vi "Main.vi"() -> ()   [LabVIEW 2020]
doc: "This template is for the Queued Message Handler design pattern.\n\nThe Event Handling Loop generates messages based on user interface actions.\n\nThe Message Handling Loop processes messages generated by the Event Handling Loop, or by other messages. The messages are string values, so new messages can be added easily to the Message Cases case structure in the Message Handling Loop. Each message cluster can also provide an optional value for Message Data, which is a variant that can be converted to whatever message-specific data is required."
uses:
  controls/UI Data.ctl
  support/Message Queue/Enqueue Message (Single).vi
  <vilib>/Utility/error.llb/Error Cluster From Error Code.vi
  <vilib>/ErrorRing/Error Ring.xnode
  support/Message Queue/Message Queue.lvlib
  support/User Event - Stop/User Event - Stop.lvlib
panel:
  out "Status":bool
  out "Wybrany zakres f":string
  in  "Pojemnik":enum32{"Page 1", "Page 2"}(tab)
  in  "Kondensator 1":bool
  in  "Kondensator 2":bool
  in  "Kondensator 3":bool
  in  "Kondensator 4":bool
  in  "Cewka":bool
  in  "Cewki":enum32{"Cewki", "Page 2"}(tab)
  in  "L1":bool
  in  "L2":bool
  in  "L 3":bool
  in  "L 4":bool
  in  "Zakres Q":u8(knob) scale=0.0..10.0
  in  "C_reg2":dbl(knob) scale=-5.0..5.0
  in  "Zakres f":u8(knob) scale=0.0..6.0
  in  "ON/OFF":bool
  out "Dobroæ":dbl(knob) scale=0.0..50.0
  in  "C_reg":dbl(knob) scale=520.0..30.0
  in  "Czêstotliwoœæ":dbl(knob) min=3.0 max=950.0 scale=950.0..1045.0
  in  "Exit":bool
  # "Q"
  # "f"
  # "C (pF)"
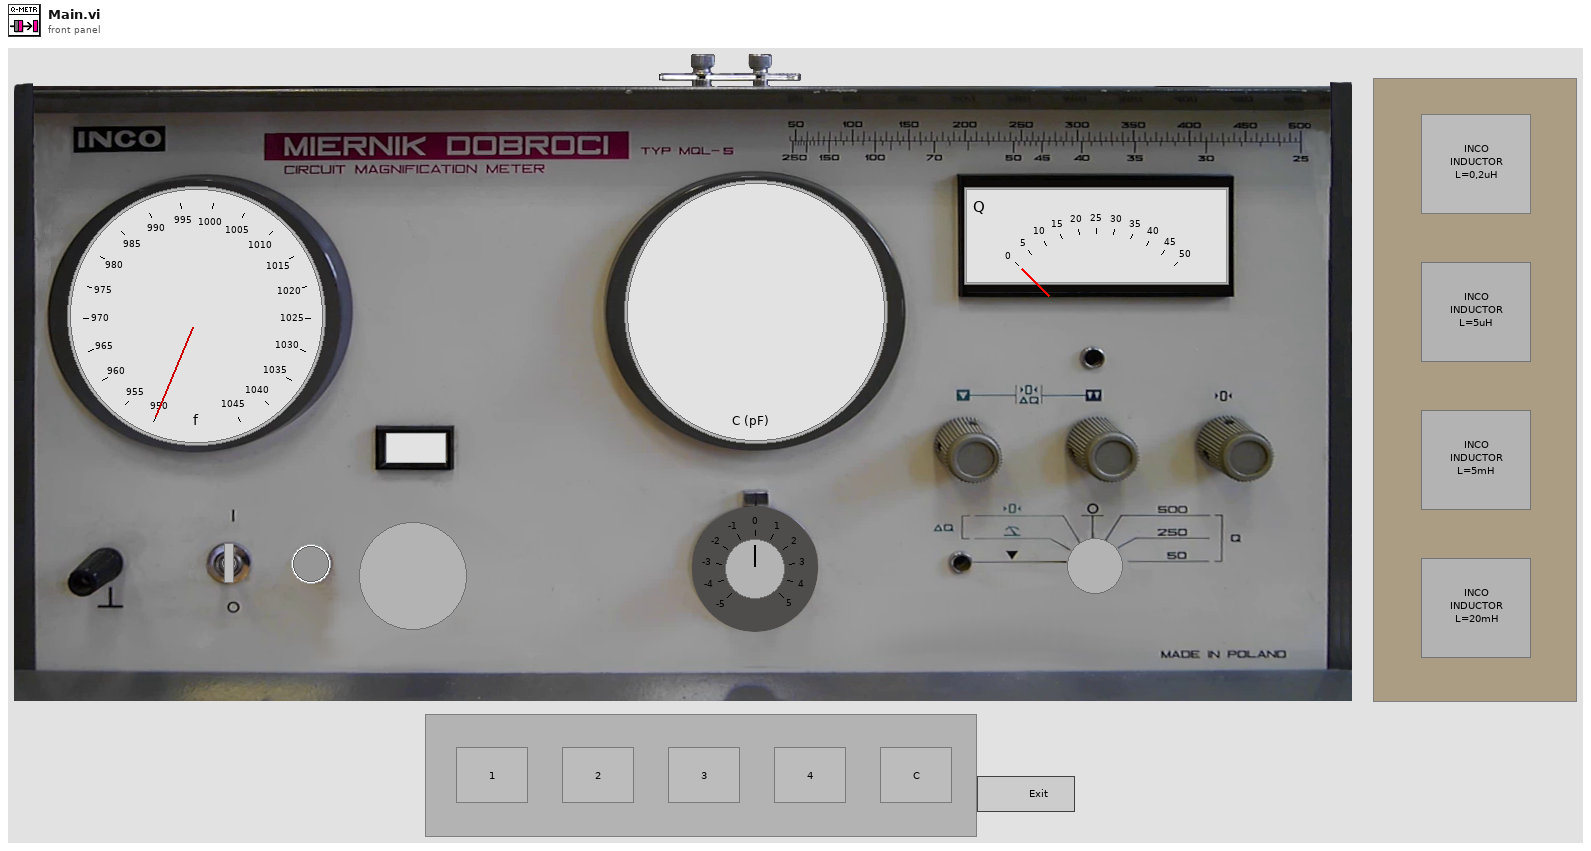
[diagram p1: front panel]
types:
  T1 = typedef "UI Data.ctl" = cluster{"Zakres freq":u8, "Status":bool, "C_reg":dbl, "C_reg2":dbl, "L1":bool, "L2":bool, "L3":bool, "L4":bool, "L value":dbl, "C1":bool, "C2":bool, "C3":bool, "C4":bool, "C measure":dbl, "Freq":dbl, "Q elementu":dbl, "L cewka":bool, "C prev":dbl, "C byl zamon.":bool, "Q prev":dbl}
  T2 = typedef "Message Queue.lvlib/All Message Queues.ctl" = cluster{"UI":refnum<queue>}
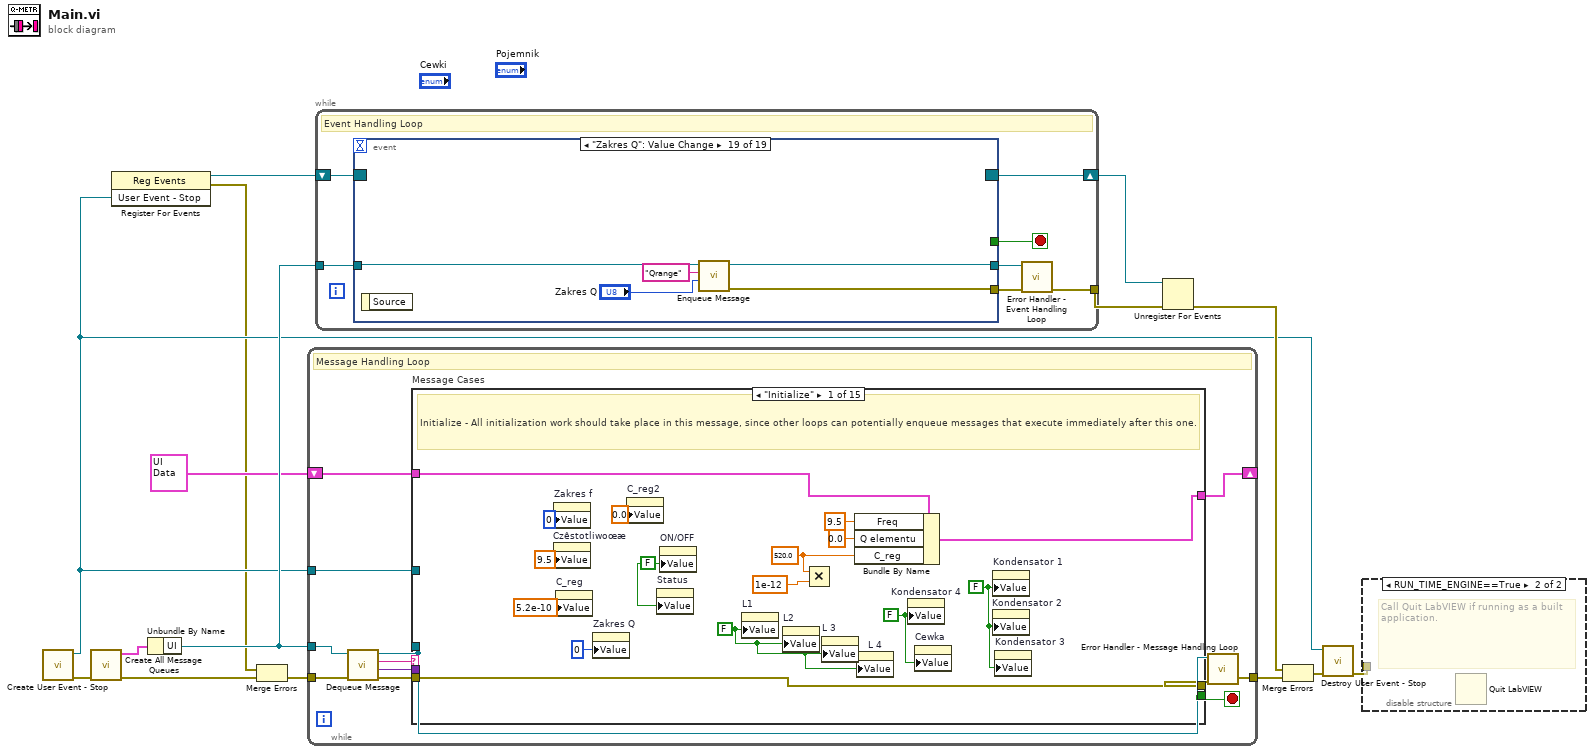
[diagram p0: block diagram]
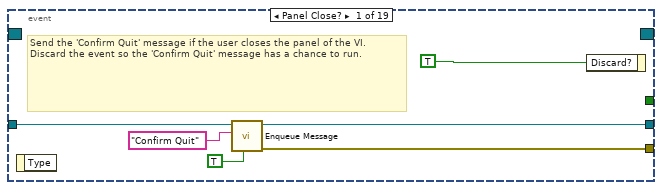
[diagram p3: hidden frame]
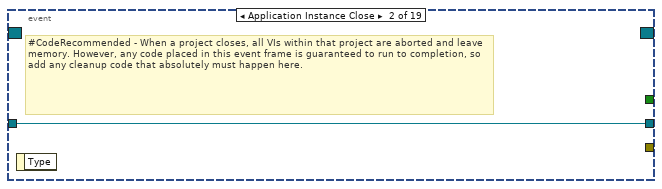
[diagram p4: hidden frame]
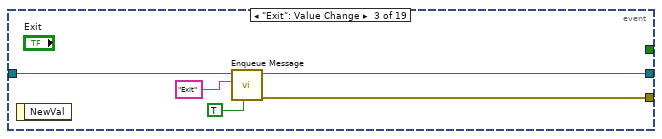
[diagram p5: hidden frame]
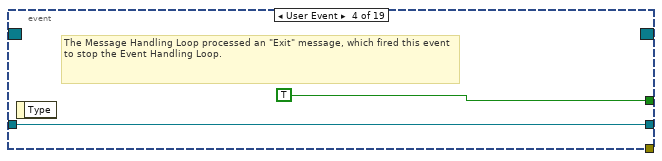
[diagram p6: hidden frame]
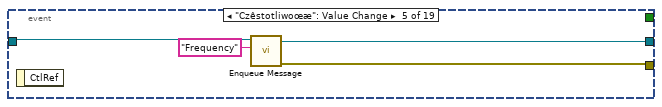
[diagram p7: hidden frame]
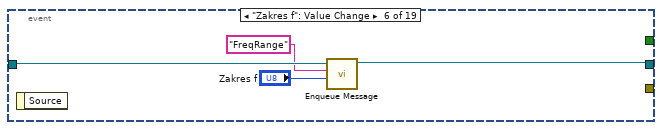
[diagram p8: hidden frame]
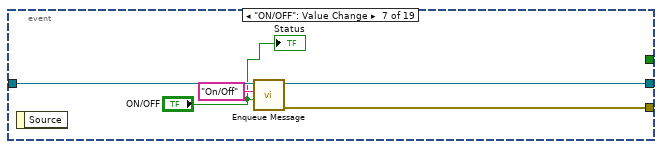
[diagram p9: hidden frame]
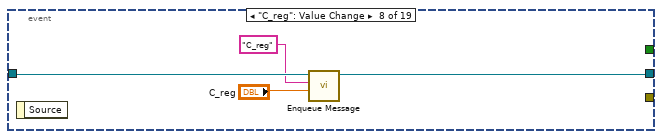
[diagram p10: hidden frame]
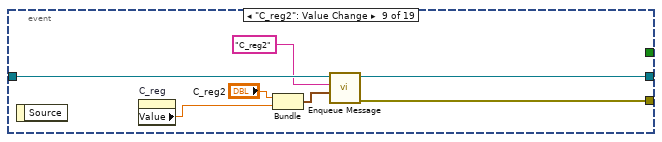
[diagram p11: hidden frame]
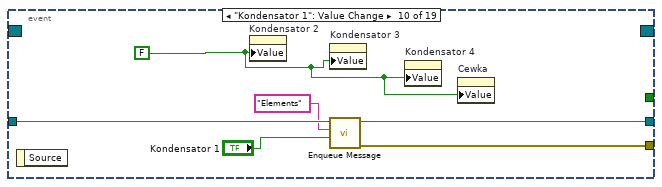
[diagram p12: hidden frame]
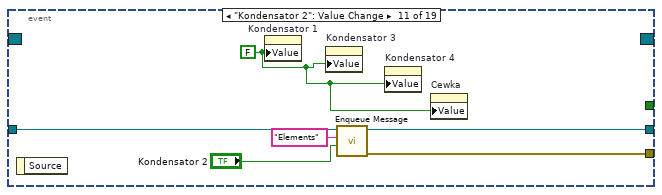
[diagram p13: hidden frame]
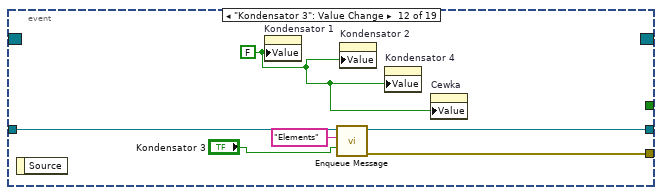
[diagram p14: hidden frame]
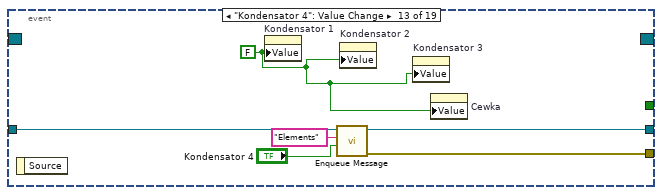
[diagram p15: hidden frame]
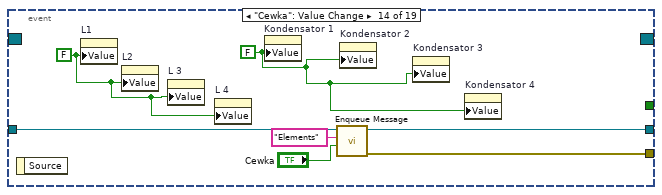
[diagram p16: hidden frame]
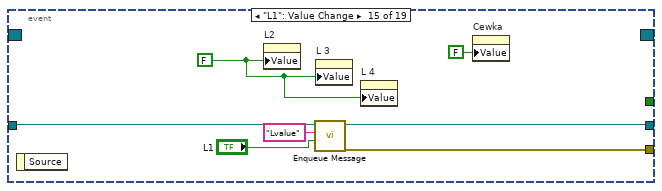
[diagram p17: hidden frame]
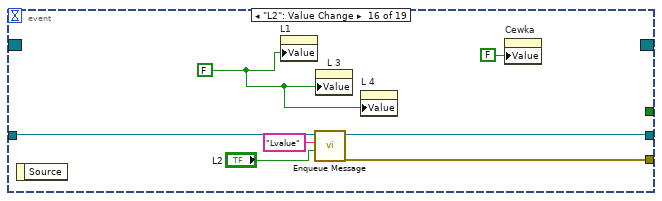
[diagram p18: hidden frame]
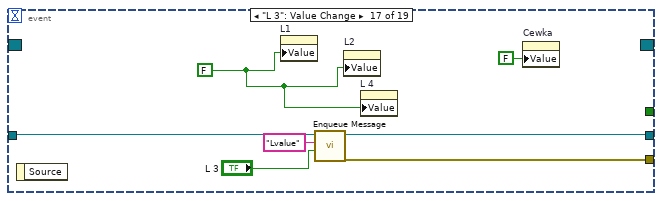
[diagram p19: hidden frame]
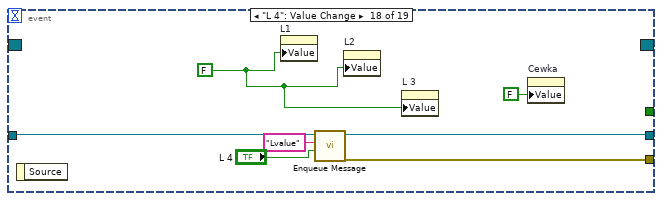
[diagram p20: hidden frame]
diagram:
  n1 = call "Create User Event - Stop.vi"() -> ("error out"=w11:errorcluster, "User Event - Stop"=w3:refnum<user-event>)  [unwired: 10 in]
  n2 = call "Create All Message Queues.vi"("error in (no error)"=w11) -> ("error out"=w15:errorcluster, "Message Queues out"=w14:T2)  [unwired: 9 in]
  n3 = register-events(w3) -> (reference out=w4:refnum<event-registration>, error out=w1:errorcluster)  [unwired: 2 in]
  n4 = Unbundle By Name(w14) -> ("UI"=w12:refnum<queue>)
  n5 = Merge Errors(w1, w15) -> (w2:errorcluster)
  n6 = while {
    tunnel: w12 -> [w20]
    shift-right: [w27] -> _
    shift-left: T1 {"Zakres freq"=0, "Status"=FALSE, "C_reg"=0.0, "C_reg2"=0.0, "L1"=FALSE, "L2"=FALSE, "L3"=FALSE, "L4"=FALSE, "L value"=0.0, "C1"=FALSE, "C2"=FALSE, "C3"=FALSE, "C4"=FALSE, "C measure"=0.0, "Freq"=0.0, "Q elementu"=0.0, "L cewka"=FALSE, "C prev"=0.0, "C byl zamon."=FALSE, "Q prev"=0.0} ("Data Cluster") -> [w16]
    tunnel: w3 -> [w25]
    tunnel: w2 -> [w24]
    tunnel: [w18] -> w13
    stop <- w26 stop-if-true
    # "Message Handling Loop"
    n7 = call "Dequeue Message.vi"("error in (no error)"=w24, "Message Queue"=w20) -> ("error out"=w23:errorcluster, "Message Data"=w21:variant, "Message"=w22:string, "dup Message Queue"=w19:refnum<queue>)  [unwired: 6 in]
    n8 = case "Message Cases" shown="\"Initialize\"" w22 {
      selector: w22 -> [_ _ _ _ _ _ _ _ _ _ _ _ _ _ w264]
      tunnel: w19 -> [_ _ w53 _ w66 w80 w110 w163 w175 w188 w218 w233 _ w263 _]
      tunnel: w23 -> [w43 w50 w57 w60 w68 w79 w111 w165 w177 w186 w217 w235 w252 w256 _]
      tunnel: [w43 w44 w55 w58 w69 w81 w113 w166 w178 w189 w220 w236 w251 w259 w265] -> w17
      tunnel: w16 -> [w37 w49 w56 w59 w70 w76 w107 w157 w171 w182 w216 w229 w250 w262 w266]
      tunnel: [w36 w49 w56 w59 w70 w75 w106 w161 w170 w180 w216 w228 w250 w262 w266] -> w27
      tunnel: [_ _ _ _ _ _ _ _ _ _ _ _ _ TRUE _] -> w26
      tunnel: w21 -> [_ w48 _ _ w64 _ _ w160 w173 w184 _ _ _ w253 _]
      tunnel: w25 -> [_ _ _ _ _ _ _ _ _ _ _ _ _ w258 _]
      frame "Initialize" {
        w29 = FALSE ("L1")
        w30 = FALSE ("Kondensator 4")
        w31 = FALSE ("Kondensator 1")
        w33 = 520.0 ("C_reg")
        w38 = FALSE ("ON/OFF")
        # "Initialize - All initialization work should take place in this message, since other loops can potentially enqueue messages that execute immediately after this one."
        n9 = property on="Zakres f" class="Knob (strict)"("Value"=u8 0 ("Zakres f")) -> ()  [unwired: 2 in, 2 out]
        n10 = property on="Czêstotliwoœæ" class="Knob (strict)"("Value"=9.5 ("Czêstotliwoœæ")) -> ()  [unwired: 2 in, 2 out]
        n11 = property on="C_reg" class="Knob (strict)"("Value"=5.2e-10 ("C_reg")) -> ()  [unwired: 2 in, 2 out]
        n12 = property on="Zakres Q" class="Knob (strict)"("Value"=u8 0 ("Zakres Q")) -> ()  [unwired: 2 in, 2 out]
        n13 = property on="C_reg2" class="Knob (strict)"("Value"=0.0 ("C_reg2")) -> ()  [unwired: 2 in, 2 out]
        n14 = property on="Status" class="Bool (strict)"("Value"=w38) -> ()  [unwired: 2 in, 2 out]
        n15 = property on="ON/OFF" class="Bool (strict)"("Value"=w38) -> ()  [unwired: 2 in, 2 out]
        n16 = property on="L1" class="Bool (strict)"("Value"=w29) -> ()  [unwired: 2 in, 2 out]
        n17 = property on="L2" class="Bool (strict)"("Value"=w29) -> ()  [unwired: 2 in, 2 out]
        n18 = Multiply(x=w33, y=1e-12) -> ()  [unwired: 1 out]
        n19 = property on="L 3" class="Bool (strict)"("Value"=w29) -> ()  [unwired: 2 in, 2 out]
        n20 = Bundle By Name(cluster=w37, "Freq"=9.5, "Q elementu"=0.0, "C_reg"=w33) -> (w36:T1)
        n21 = property on="L 4" class="Bool (strict)"("Value"=w29) -> ()  [unwired: 2 in, 2 out]
        n22 = property on="Kondensator 4" class="Bool (strict)"("Value"=w30) -> ()  [unwired: 2 in, 2 out]
        n23 = property on="Cewka" class="Bool (strict)"("Value"=w30) -> ()  [unwired: 2 in, 2 out]
        n24 = property on="Kondensator 1" class="Bool (strict)"("Value"=w31) -> ()  [unwired: 2 in, 2 out]
        n25 = property on="Kondensator 2" class="Bool (strict)"("Value"=w31) -> ()  [unwired: 2 in, 2 out]
        n26 = property on="Kondensator 3" class="Bool (strict)"("Value"=w31) -> ()  [unwired: 2 in, 2 out]
      }
      frame "Error" {
        # "#CodeRecommended - If you ever change the name of this \"Error\" message, you'll need to update the name in the Check Loop Error.vi as well."
        # "#CodeRecommended - Consider creating a system for logging errors in some way. These errors are for notification purposes only. Handling of specific errors should be performed in the message frames that generated the error."
        # "Error - Display an error dialog. This message is sent by the \"Error Handler\" VIs at the end of other loops in this application."
        n27 = Variant To Data(error in=w50, type=errorcluster {"status"=FALSE, "code"=0, "source"=""} ("error constant"), Variant=w48) -> (data=w46:errorcluster, error out=w45:errorcluster)
        n28 = call <vilib>:"Simple Error Handler.vi"("error in (no error)"=w46) -> ()  [unwired: 4 in, 5 out]
        n29 = Merge Errors(w45) -> (w44:errorcluster)
      }
      frame "Confirm Quit" {
        # "#CodeNeeded - If you want to provide an \"Are you sure\" dialog (or some other notification) before the application exits, place that code here. This message is typically sent from a Panel Close? event."
        # "Confirm Quit - Message that can confirm whether or not the user wants to exit the application."
        n30 = call-poly "Enqueue Message.vi"("Priority Message? (F)"=TRUE, "error in (no error)"=w57, "Message"="Exit", "Message Queue"=w53) -> ("error out"=w54:errorcluster)  [unwired: 6 in, 1 out]
        n31 = Merge Errors(w54) -> (w55:errorcluster)
      }
      frame "---Copy This Frame---" {
        # "Duplicate this frame when creating new messages.  Change this comment in the duplicated frame to describe this message."
        n32 = Merge Errors(w60) -> (w58:errorcluster)
      }
      frame "Qrange" {
        # "Duplicate this frame when creating new messages.  Change this comment in the duplicated frame to describe this message."
        n33 = Variant To Data(type=u8 0 ("Zakres Q"), Variant=w64) -> (data=w62:u8)  [unwired: 1 in, 1 out]
        n34 = call-poly "Enqueue Message.vi"("error in (no error)"=w68, "Message"="On/Off", "Message Queue"=w66) -> ("error out"=w67:errorcluster)  [unwired: 7 in, 1 out]
        n35 = case shown="8.." w62 {
          tunnel: [500.0 ("Scale.Range:Maximum") 250.0 ("Scale.Range:Maximum") 50.0 ("Scale.Range:Maximum")] -> w61
          frame 0..6, Default {
          }
          frame 7 {
          }
          frame 8.. {
          }
        }
        n36 = property on="Dobroæ" class="Knob (strict)"("Scale.Maximum"=w61) -> ()  [unwired: 2 in, 2 out]
        n37 = Merge Errors(w67) -> (w69:errorcluster)
      }
      frame "Lvalue" {
        # "Duplicate this frame when creating new messages.  Change this comment in the duplicated frame to describe this message."
        n38 = property on="L1" class="Bool (strict)"() -> ("Value"=w74:bool)  [unwired: 2 in, 2 out]
        n39 = call-poly "Enqueue Message.vi"("error in (no error)"=w79, "Message"="On/Off", "Message Queue"=w80) -> ("error out"=w78:errorcluster)  [unwired: 7 in, 1 out]
        n40 = case shown="False" w74 {
          tunnel: w76 -> [w83 w105]
          tunnel: [w82 w104] -> w75
          frame False {
            n41 = property on="L2" class="Bool (strict)"() -> ("Value"=w84:bool)  [unwired: 2 in, 2 out]
            n42 = case shown="False" w84 {
              tunnel: w83 -> [w86 w102]
              tunnel: [w85 w101] -> w82
              frame False {
                n43 = property on="L 3" class="Bool (strict)"() -> ("Value"=w87:bool)  [unwired: 2 in, 2 out]
                n44 = case shown="False" w87 {
                  tunnel: w86 -> [w89 w99]
                  tunnel: [w88 w98] -> w85
                  frame False {
                    n45 = property on="L 4" class="Bool (strict)"() -> ("Value"=w90:bool)  [unwired: 2 in, 2 out]
                    n46 = case shown="False" w90 {
                      tunnel: w89 -> [w93 w96]
                      tunnel: [w92 w95] -> w88
                      frame False {
                        n47 = Bundle By Name(cluster=w93, "L value"=0.0) -> (w92:T1)
                      }
                      frame True {
                        n48 = Bundle By Name(cluster=w96, "L value"=0.02) -> (w95:T1)
                      }
                    }
                  }
                  frame True {
                    n49 = Bundle By Name(cluster=w99, "L value"=0.005) -> (w98:T1)
                  }
                }
              }
              frame True {
                n50 = Bundle By Name(cluster=w102, "L value"=5e-06) -> (w101:T1)
              }
            }
          }
          frame True {
            n51 = Bundle By Name(cluster=w105, "L value"=2e-07) -> (w104:T1)
          }
        }
        n52 = Merge Errors(w78) -> (w81:errorcluster)
      }
      frame "Elements" {
        # "Duplicate this frame when creating new messages.  Change this comment in the duplicated frame to describe this message."
        n53 = property on="Kondensator 1" class="Bool (strict)"() -> ("Value"=w108:bool)  [unwired: 2 in, 2 out]
        n54 = case shown="True" w108 {
          tunnel: w107 -> [w115 w149]
          tunnel: [w114 w148] -> w106
          frame False {
            n55 = property on="Kondensator 2" class="Bool (strict)"() -> ("Value"=w116:bool)  [unwired: 2 in, 2 out]
            n56 = case shown="True" w116 {
              tunnel: w115 -> [w119 w145]
              tunnel: [w118 w144] -> w114
              frame False {
                n57 = property on="Kondensator 3" class="Bool (strict)"() -> ("Value"=w117:bool)  [unwired: 2 in, 2 out]
                n58 = case shown="False" w117 {
                  tunnel: w119 -> [w121 w141]
                  tunnel: [w120 w140] -> w118
                  frame False {
                    n59 = property on="Kondensator 4" class="Bool (strict)"() -> ("Value"=w122:bool)  [unwired: 2 in, 2 out]
                    n60 = case shown="False" w122 {
                      tunnel: w121 -> [w124 w137]
                      tunnel: [w123 w136] -> w120
                      frame False {
                        n61 = property on="Cewka" class="Bool (strict)"() -> ("Value"=w125:bool)  [unwired: 2 in, 2 out]
                        n62 = case shown="False" w125 {
                          tunnel: w124 -> [w128 w133]
                          tunnel: [w129 w132] -> w123
                          frame False {
                            n63 = Bundle By Name(cluster=w128, "Q elementu"=0.0, "C measure"=0.0) -> (w129:T1)
                          }
                          frame True {
                            n64 = Bundle By Name(cluster=w133, "Q elementu"=42.0, "C measure"=6.47e-05) -> (w132:T1)
                          }
                        }
                      }
                      frame True {
                        n65 = Bundle By Name(cluster=w137, "Q elementu"=239.0, "C measure"=1.2e-10) -> (w136:T1)
                      }
                    }
                  }
                  frame True {
                    n66 = Bundle By Name(cluster=w141, "Q elementu"=73.0, "C measure"=2.19e-09) -> (w140:T1)
                  }
                }
              }
              frame True {
                n67 = Bundle By Name(cluster=w145, "Q elementu"=277.0, "C measure"=1.03e-10) -> (w144:T1)
              }
            }
          }
          frame True {
            n68 = Bundle By Name(cluster=w149, "Q elementu"=310.0, "C measure"=9.99e-09) -> (w148:T1)
          }
        }
        n69 = call-poly "Enqueue Message.vi"("error in (no error)"=w111, "Message"="On/Off", "Message Queue"=w110) -> ("error out"=w112:errorcluster)  [unwired: 7 in, 1 out]
        n70 = Merge Errors(w112) -> (w113:errorcluster)
      }
      frame "C_reg2" {
        # "Duplicate this frame when creating new messages.  Change this comment in the duplicated frame to describe this message."
        n71 = Variant To Data(type=cluster{dbl, dbl} {0.0, 0.0}, Variant=w160) -> (data=w158:cluster{dbl, dbl})  [unwired: 1 in, 1 out]
        n72 = Unbundle By Name(w157) -> ("C_reg2"=w155:dbl)
        n73 = call-poly "Enqueue Message.vi"("error in (no error)"=w165, "Message"="On/Off", "Message Queue"=w163) -> ("error out"=w164:errorcluster)  [unwired: 7 in, 1 out]
        n74 = Unbundle(w158) -> (w153:dbl, w156:dbl)
        n75 = Subtract(x=w156, y=w155) -> (x-y=w154:dbl)
        n76 = Add(x=w154, y=w153) -> (x+y=w152:dbl)
        n77 = Multiply(x=1e-12, y=w152) -> (x*y=w150:dbl)
        n78 = local write "C_reg"(w152) -> ()
        n79 = Merge Errors(w164) -> (w166:errorcluster)
        n80 = Bundle By Name(cluster=w157, "C_reg2"=w153, "C_reg"=w150) -> (w161:T1)
      }
      frame "C_reg" {
        # "Duplicate this frame when creating new messages.  Change this comment in the duplicated frame to describe this message."
        n81 = Variant To Data(type=0.0, Variant=w173) -> (data=w169:dbl)  [unwired: 1 in, 1 out]
        n82 = call-poly "Enqueue Message.vi"("error in (no error)"=w177, "Message"="On/Off", "Message Queue"=w175) -> ("error out"=w176:errorcluster)  [unwired: 7 in, 1 out]
        n83 = Multiply(x=w169, y=1e-12) -> (x*y=w168:dbl)
        n84 = Bundle By Name(cluster=w171, "C_reg"=w168) -> (w170:T1)
        n85 = Merge Errors(w176) -> (w178:errorcluster)
      }
      frame "FreqRange" {
        # "Duplicate this frame when creating new messages.  Change this comment in the duplicated frame to describe this message."
        n86 = Variant To Data(type=0, Variant=w184) -> (data=w181:i32)  [unwired: 1 in, 1 out]
        n87 = call-poly "Enqueue Message.vi"("error in (no error)"=w186, "Message"="Frequency", "Message Queue"=w188) -> ("error out"=w187:errorcluster)  [unwired: 7 in, 1 out]
        n88 = Bundle By Name(cluster=w182, "Zakres freq"=w181) -> (w180:T1)
        n89 = property on="Status" class="Bool (strict)"() -> ("Value"=w179:bool)  [unwired: 2 in, 2 out]
        n90 = case shown="True" w179 {
          tunnel: w181 -> [_ w193]
          frame False {
          }
          frame True {
            n91 = case shown="1" w193 {
              tunnel: [30.0 ("Scale.Range:Maximum") 95.0 ("Scale.Range:Maximum") 300.0 ("Scale.Range:Maximum") 950.0 ("Scale.Range:Maximum") 3.0 ("Scale.Range:Maximum") 9.5 ("Scale.Range:Maximum") 30.0 ("Scale.Range:Maximum")] -> w192
              tunnel: [95.0 ("Scale.Range:Minimum") 300.0 ("Scale.Range:Minimum") 950.0 ("Scale.Range:Minimum") 3000.0 ("Scale.Range:Minimum") 9.5 ("Scale.Range:Minimum") 30.0 ("Scale.Range:Minimum") 75.0 ("Scale.Range:Minimum")] -> w191
              tunnel: ["30-95 kHz" ("Wybrany zakres f") "95-300 kHz" ("Wybrany zakres f") "300-950 kHz" ("Wybrany zakres f") "950-3000 kHz" ("Wybrany zakres f") "3-9,5 MHz" ("Wybrany zakres f") "9,5-30 MHz" ("Wybrany zakres f") "30-75 MHz" ("Wybrany zakres f")] -> w190
              frame 0, Default {
              }
              frame 1 {
              }
              frame 2 {
              }
              frame 3 {
              }
              frame 4 {
              }
              frame 5 {
              }
              frame 6 {
              }
            }
            "Wybrany zakres f" <- w190
            n92 = property on="Czêstotliwoœæ" class="Knob (strict)"("Scale.Maximum"=w192, "Scale.Minimum"=w191) -> ()  [unwired: 2 in, 2 out]
          }
        }
        n93 = Merge Errors(w187) -> (w189:errorcluster)
      }
      frame "On/Off" {
        # "Duplicate this frame when creating new messages.  Change this comment in the duplicated frame to describe this message."
        n94 = property on="Status" class="Bool (strict)"() -> ("Value"=w215:bool)  [unwired: 2 in, 2 out]
        n95 = case shown="True" w215 {
          tunnel: [w221 w225] -> w219
          tunnel: w218 -> [_ w224]
          tunnel: w217 -> [w221 w223]
          frame False {
          }
          frame True {
            n96 = call-poly "Enqueue Message.vi"("error in (no error)"=w223, "Message"="Calculate Q", "Message Queue"=w224) -> ("error out"=w225:errorcluster)  [unwired: 7 in, 1 out]
          }
        }
        n97 = Merge Errors(w219) -> (w220:errorcluster)
      }
      frame "Frequency" {
        # "Duplicate this frame when creating new messages.  Change this comment in the duplicated frame to describe this message."
        n98 = Unbundle By Name(w229) -> ("Zakres freq"=w231:u8)
        n99 = call-poly "Enqueue Message.vi"("error in (no error)"=w235, "Message"="On/Off", "Message Queue"=w233) -> ("error out"=w234:errorcluster)  [unwired: 7 in, 1 out]
        n100 = case shown="0..3, Default" w231 {
          tunnel: [1000.0 1000000.0] -> w230
          frame 0..3, Default {
          }
          frame 4..6 {
          }
        }
        n101 = Multiply(x=w230, y="Czêstotliwoœæ") -> (x*y=w227:dbl)
        n102 = Bundle By Name(cluster=w229, "Freq"=w227) -> (w228:T1)
        n103 = Merge Errors(w234) -> (w236:errorcluster)
      }
      frame "Calculate Q" {
        # "Calculate the Q value."
        n104 = Unbundle By Name(w250) -> ("Q elementu"=w240:dbl, "C measure"=w244:dbl, "C_reg"=w243:dbl, "L value"=w242:dbl)
        n105 = call "Cz.vi"("C_reg"=w243, "C"=w244) -> ("Cz"=w245:dbl)  [unwired: 9 in]
        n106 = call "frez.vi"("Cz"=w245, "L"=w242) -> ("f_rez"=w239:dbl)  [unwired: 9 in]
        n107 = call "I.vi"("Q"=w240, "C_reg"=w243, "C"=w244, "L"=w242, "f"=w239) -> ("I"=w247:dbl)  [unwired: 6 in]
        n108 = Unbundle By Name(w250) -> ("Freq"=w241:dbl)
        n109 = call "I.vi"("Q"=w240, "C_reg"=w243, "C"=w244, "L"=w242, "f"=w241) -> ("I"=w246:dbl)  [unwired: 6 in]
        n110 = Merge Errors(w252) -> (w251:errorcluster)
        n111 = Divide(x=w246, y=w247) -> (x/y=w248:dbl)
        n112 = Multiply(x=w240, y=w248) -> (x*y=→"Dobroæ":dbl)
      }
      frame "Exit" {
        # "Stop the VI"
        # "Release the message queue reference"
        # "#CodeNeeded - Add any required cleanup code here. Note that if 'Exit' was called as a result of an error, an error dialog will be displayed. Add any custom error handling for an 'Exit' condition here as well."
        # "Exit - Exit the application."
        n113 = Variant To Data(type=errorcluster {"status"=FALSE, "code"=0, "source"=""} ("error constant"), Variant=w253) -> (data=w254:errorcluster)  [unwired: 1 in, 1 out]
        n114 = call <vilib>:"Simple Error Handler.vi"("error in (no error)"=w254) -> ()  [unwired: 4 in, 5 out]
        n115 = call "Fire User Event - Stop.vi"("User Event - Stop"=w258) -> ("error out"=w257:errorcluster)  [unwired: 10 in]
        n116 = Release Queue(queue=w263, error in (no error)=w256) -> (error out=w260:errorcluster)  [unwired: 1 in, 2 out]
        n117 = Merge Errors(w257, w260) -> (w259:errorcluster)
      }
      frame Default {
        # "'Default' case only runs if there is a message that isn't defined in any of the other cases.  Output a programming error."
        n118 = xnode "Error Ring"("parameter 0"=w264) -> ("error out"=w265:errorcluster)
      }
    }
    n119 = call "Error Handler - Message Handling Loop.vi"("error in (no error)"=w17, "Message Queue"=w19) -> ("dup error in"=w18:errorcluster)  [unwired: 8 in, 1 out]
  }
  n120 = while {
    tunnel: w12 -> [w280]
    shift-right: [w278] -> w8
    shift-left: w4 -> [w279]
    tunnel: [w274] -> w5
    stop <- w276 stop-if-true
    # "Event Handling Loop"
    n121 = event shown="[18] \"Zakres Q\": Value Change" {
      selector: w279 -> [_ _ _ _ _ _ _ _ _ _ _ _ _ _ _ _ _ _ _]
      dyn-events: [_ _ _ _ _ _ _ _ _ _ _ _ _ _ _ _ _ _ _] -> w278
      timeout: _ -> [_ _ _ _ _ _ _ _ _ _ _ _ _ _ _ _ _ _ _]
      tunnel: [_ _ _ TRUE ("Discard?") _ _ _ _ _ _ _ _ _ _ _ _ _ _ _] -> w276
      tunnel: w280 -> [w285 w287 w292 w294 w298 w302 w307 w311 w318 w324 w330 w336 w342 w349 w356 w363 w370 w377 w382]
      tunnel: [w284 _ w291 _ w296 _ w305 _ w312 w322 w329 w335 w341 w348 w354 w361 w368 w375 w380] -> w277
      tunnel: [w283 w287 w290 w294 w297 w301 w306 w310 w317 w323 w328 w334 w340 w347 w355 w362 w369 w376 w381] -> w275
      event Panel Close? {
        # "Send the 'Confirm Quit' message if the user closes the panel of the VI. Discard the event so the 'Confirm Quit' message has a chance to run."
        n122 = event-data() -> ()  [unwired: 1 in, 1 out]
        n123 = call-poly "Enqueue Message.vi"("Priority Message? (F)"=TRUE, "Message"="Confirm Quit", "Message Queue"=w285) -> ("error out"=w284:errorcluster, "dup Message Queue"=w283:refnum<queue>)  [unwired: 7 in]
        n124 = event-data("Discard?"=TRUE) -> ()  [unwired: 1 in, 1 out]
      }
      event Application Instance Close {
        # "#CodeRecommended - When a project closes, all VIs within that project are aborted and leave memory. However, any code placed in this event frame is guaranteed to run to completion, so add any cleanup code that absolutely must happen here."
        n125 = event-data() -> ()  [unwired: 1 in, 1 out]
      }
      event "Exit": Value Change {
        n126 = event-data() -> ()  [unwired: 1 in, 1 out]
        n127 = call-poly "Enqueue Message.vi"("Priority Message? (F)"=TRUE, "Message"="Exit", "Message Queue"=w292) -> ("error out"=w291:errorcluster, "dup Message Queue"=w290:refnum<queue>)  [unwired: 7 in]
      }
      event User Event {
        # "The Message Handling Loop processed an \"Exit\" message, which fired this event to stop the Event Handling Loop."
        n128 = event-data() -> ()  [unwired: 1 in, 1 out]
      }
      event "Czêstotliwoœæ": Value Change {
        n129 = event-data() -> ()  [unwired: 1 in, 1 out]
        n130 = call-poly "Enqueue Message.vi"("Message"="Frequency", "Message Queue"=w298) -> ("error out"=w296:errorcluster, "dup Message Queue"=w297:refnum<queue>)  [unwired: 8 in]
      }
      event "Zakres f": Value Change {
        n131 = event-data() -> ()  [unwired: 1 in, 1 out]
        n132 = call-poly "Enqueue Message.vi"("Message Data"="Zakres f", "Message"="FreqRange", "Message Queue"=w302) -> ("dup Message Queue"=w301:refnum<queue>)  [unwired: 7 in, 1 out]
      }
      event "ON/OFF": Value Change {
        n133 = event-data() -> ()  [unwired: 1 in, 1 out]
        n134 = call-poly "Enqueue Message.vi"("Message Data"="ON/OFF", "Message"="On/Off", "Message Queue"=w307) -> ("error out"=w305:errorcluster, "dup Message Queue"=w306:refnum<queue>)  [unwired: 7 in]
        "Status" <- "ON/OFF"
      }
      event "C_reg": Value Change {
        n135 = event-data() -> ()  [unwired: 1 in, 1 out]
        n136 = call-poly "Enqueue Message.vi"("Message Data"="C_reg", "Message"="C_reg", "Message Queue"=w311) -> ("dup Message Queue"=w310:refnum<queue>)  [unwired: 7 in, 1 out]
      }
      event "C_reg2": Value Change {
        n137 = event-data() -> ()  [unwired: 1 in, 1 out]
        n138 = property on="C_reg" class="Knob (strict)"() -> ("Value"=w314:dbl)  [unwired: 2 in, 2 out]
        n139 = Bundle("C_reg2"="C_reg2", "Value"=w314) -> (w313:cluster{"C_reg2":dbl, "Value":dbl})  [unwired: 1 in]
        n140 = call-poly "Enqueue Message.vi"("Message Data"=w313, "Message"="C_reg2", "Message Queue"=w318) -> ("error out"=w312:errorcluster, "dup Message Queue"=w317:refnum<queue>)  [unwired: 7 in]
      }
      event "Kondensator 1": Value Change {
        w320 = FALSE ("Kondensator 2")
        n141 = event-data() -> ()  [unwired: 1 in, 1 out]
        n142 = property on="Kondensator 2" class="Bool (strict)"("Value"=w320) -> ()  [unwired: 2 in, 2 out]
        n143 = property on="Kondensator 3" class="Bool (strict)"("Value"=w320) -> ()  [unwired: 2 in, 2 out]
        n144 = call-poly "Enqueue Message.vi"("Message Data"="Kondensator 1", "Message"="Elements", "Message Queue"=w324) -> ("error out"=w322:errorcluster, "dup Message Queue"=w323:refnum<queue>)  [unwired: 7 in]
        n145 = property on="Kondensator 4" class="Bool (strict)"("Value"=w320) -> ()  [unwired: 2 in, 2 out]
        n146 = property on="Cewka" class="Bool (strict)"("Value"=w320) -> ()  [unwired: 2 in, 2 out]
      }
      event "Kondensator 2": Value Change {
        w326 = FALSE ("Kondensator 1")
        n147 = event-data() -> ()  [unwired: 1 in, 1 out]
        n148 = property on="Kondensator 1" class="Bool (strict)"("Value"=w326) -> ()  [unwired: 2 in, 2 out]
        n149 = property on="Kondensator 3" class="Bool (strict)"("Value"=w326) -> ()  [unwired: 2 in, 2 out]
        n150 = call-poly "Enqueue Message.vi"("Message Data"="Kondensator 2", "Message"="Elements", "Message Queue"=w330) -> ("error out"=w329:errorcluster, "dup Message Queue"=w328:refnum<queue>)  [unwired: 7 in]
        n151 = property on="Kondensator 4" class="Bool (strict)"("Value"=w326) -> ()  [unwired: 2 in, 2 out]
        n152 = property on="Cewka" class="Bool (strict)"("Value"=w326) -> ()  [unwired: 2 in, 2 out]
      }
      event "Kondensator 3": Value Change {
        w332 = FALSE ("Kondensator 1")
        n153 = event-data() -> ()  [unwired: 1 in, 1 out]
        n154 = property on="Kondensator 1" class="Bool (strict)"("Value"=w332) -> ()  [unwired: 2 in, 2 out]
        n155 = call-poly "Enqueue Message.vi"("Message Data"="Kondensator 3", "Message"="Elements", "Message Queue"=w336) -> ("error out"=w335:errorcluster, "dup Message Queue"=w334:refnum<queue>)  [unwired: 7 in]
        n156 = property on="Kondensator 2" class="Bool (strict)"("Value"=w332) -> ()  [unwired: 2 in, 2 out]
        n157 = property on="Kondensator 4" class="Bool (strict)"("Value"=w332) -> ()  [unwired: 2 in, 2 out]
        n158 = property on="Cewka" class="Bool (strict)"("Value"=w332) -> ()  [unwired: 2 in, 2 out]
      }
      event "Kondensator 4": Value Change {
        w338 = FALSE ("Kondensator 1")
        n159 = event-data() -> ()  [unwired: 1 in, 1 out]
        n160 = property on="Kondensator 1" class="Bool (strict)"("Value"=w338) -> ()  [unwired: 2 in, 2 out]
        n161 = call-poly "Enqueue Message.vi"("Message Data"="Kondensator 4", "Message"="Elements", "Message Queue"=w342) -> ("error out"=w341:errorcluster, "dup Message Queue"=w340:refnum<queue>)  [unwired: 7 in]
        n162 = property on="Kondensator 2" class="Bool (strict)"("Value"=w338) -> ()  [unwired: 2 in, 2 out]
        n163 = property on="Kondensator 3" class="Bool (strict)"("Value"=w338) -> ()  [unwired: 2 in, 2 out]
        n164 = property on="Cewka" class="Bool (strict)"("Value"=w338) -> ()  [unwired: 2 in, 2 out]
      }
      event "Cewka": Value Change {
        w343 = FALSE ("L1")
        w345 = FALSE ("Kondensator 1")
        n165 = event-data() -> ()  [unwired: 1 in, 1 out]
        n166 = property on="L1" class="Bool (strict)"("Value"=w343) -> ()  [unwired: 2 in, 2 out]
        n167 = property on="L2" class="Bool (strict)"("Value"=w343) -> ()  [unwired: 2 in, 2 out]
        n168 = property on="L 3" class="Bool (strict)"("Value"=w343) -> ()  [unwired: 2 in, 2 out]
        n169 = property on="L 4" class="Bool (strict)"("Value"=w343) -> ()  [unwired: 2 in, 2 out]
        n170 = property on="Kondensator 1" class="Bool (strict)"("Value"=w345) -> ()  [unwired: 2 in, 2 out]
        n171 = call-poly "Enqueue Message.vi"("Message Data"="Cewka", "Message"="Elements", "Message Queue"=w349) -> ("error out"=w348:errorcluster, "dup Message Queue"=w347:refnum<queue>)  [unwired: 7 in]
        n172 = property on="Kondensator 2" class="Bool (strict)"("Value"=w345) -> ()  [unwired: 2 in, 2 out]
        n173 = property on="Kondensator 3" class="Bool (strict)"("Value"=w345) -> ()  [unwired: 2 in, 2 out]
        n174 = property on="Kondensator 4" class="Bool (strict)"("Value"=w345) -> ()  [unwired: 2 in, 2 out]
      }
      event "L1": Value Change {
        w352 = FALSE ("L2")
        n175 = event-data() -> ()  [unwired: 1 in, 1 out]
        n176 = property on="L2" class="Bool (strict)"("Value"=w352) -> ()  [unwired: 2 in, 2 out]
        n177 = call-poly "Enqueue Message.vi"("Message Data"="L1", "Message"="Lvalue", "Message Queue"=w356) -> ("error out"=w354:errorcluster, "dup Message Queue"=w355:refnum<queue>)  [unwired: 7 in]
        n178 = property on="L 3" class="Bool (strict)"("Value"=w352) -> ()  [unwired: 2 in, 2 out]
        n179 = property on="L 4" class="Bool (strict)"("Value"=w352) -> ()  [unwired: 2 in, 2 out]
        n180 = property on="Cewka" class="Bool (strict)"("Value"=FALSE ("Cewka")) -> ()  [unwired: 2 in, 2 out]
      }
      event "L2": Value Change {
        w359 = FALSE ("L2")
        n181 = event-data() -> ()  [unwired: 1 in, 1 out]
        n182 = property on="L1" class="Bool (strict)"("Value"=w359) -> ()  [unwired: 2 in, 2 out]
        n183 = call-poly "Enqueue Message.vi"("Message Data"="L2", "Message"="Lvalue", "Message Queue"=w363) -> ("error out"=w361:errorcluster, "dup Message Queue"=w362:refnum<queue>)  [unwired: 7 in]
        n184 = property on="L 3" class="Bool (strict)"("Value"=w359) -> ()  [unwired: 2 in, 2 out]
        n185 = property on="L 4" class="Bool (strict)"("Value"=w359) -> ()  [unwired: 2 in, 2 out]
        n186 = property on="Cewka" class="Bool (strict)"("Value"=FALSE ("Cewka")) -> ()  [unwired: 2 in, 2 out]
      }
      event "L 3": Value Change {
        w366 = FALSE ("L2")
        n187 = event-data() -> ()  [unwired: 1 in, 1 out]
        n188 = property on="L1" class="Bool (strict)"("Value"=w366) -> ()  [unwired: 2 in, 2 out]
        n189 = call-poly "Enqueue Message.vi"("Message Data"="L 3", "Message"="Lvalue", "Message Queue"=w370) -> ("error out"=w368:errorcluster, "dup Message Queue"=w369:refnum<queue>)  [unwired: 7 in]
        n190 = property on="L2" class="Bool (strict)"("Value"=w366) -> ()  [unwired: 2 in, 2 out]
        n191 = property on="L 4" class="Bool (strict)"("Value"=w366) -> ()  [unwired: 2 in, 2 out]
        n192 = property on="Cewka" class="Bool (strict)"("Value"=FALSE ("Cewka")) -> ()  [unwired: 2 in, 2 out]
      }
      event "L 4": Value Change {
        w373 = FALSE ("L2")
        n193 = event-data() -> ()  [unwired: 1 in, 1 out]
        n194 = property on="L1" class="Bool (strict)"("Value"=w373) -> ()  [unwired: 2 in, 2 out]
        n195 = call-poly "Enqueue Message.vi"("Message Data"="L 4", "Message"="Lvalue", "Message Queue"=w377) -> ("error out"=w375:errorcluster, "dup Message Queue"=w376:refnum<queue>)  [unwired: 7 in]
        n196 = property on="L2" class="Bool (strict)"("Value"=w373) -> ()  [unwired: 2 in, 2 out]
        n197 = property on="L 3" class="Bool (strict)"("Value"=w373) -> ()  [unwired: 2 in, 2 out]
        n198 = property on="Cewka" class="Bool (strict)"("Value"=FALSE ("Cewka")) -> ()  [unwired: 2 in, 2 out]
      }
      event "Zakres Q": Value Change {
        n199 = event-data() -> ()  [unwired: 1 in, 1 out]
        n200 = call-poly "Enqueue Message.vi"("Message Data"="Zakres Q", "Message"="Qrange", "Message Queue"=w382) -> ("error out"=w380:errorcluster, "dup Message Queue"=w381:refnum<queue>)  [unwired: 7 in]
      }
    }
    n201 = call "Error Handler - Event Handling Loop.vi"("error in (no error)"=w277, "Message Queue"=w275) -> ("dup error in"=w274:errorcluster)  [unwired: 8 in, 1 out]
  }
  n202 = Unregister For Events(event registration refnum=w8, error in=w5) -> (error out=w9:errorcluster)
  n203 = Merge Errors(w9, w13) -> (w10:errorcluster)
  n204 = call "Destroy User Event - Stop.vi"("error in (no error)"=w10, "User Event - Stop"=w3) -> ("error out"=w6:errorcluster)  [unwired: 9 in]
  n205 = disable-structure shown="RUN_TIME_ENGINE==True" {
    disable-tunnel: w6 -> [_ _]
    frame condition #0 (active) {
    }
    frame condition #1 {
      # "Call Quit LabVIEW if running as a built application."
      n206 = Quit LabVIEW() -> ()  [unwired: 1 in]
    }
  }
